vi "Unflatten Names.vi"   [LabVIEW 2020, in "SLSC.lvlib"]
doc: "Converts a comma-delimited list of names into an array of names. If the list contains colon-delimited ranges, they will be expanded."
uses:
  <vilib>/SLSC/SLSC.lvlib
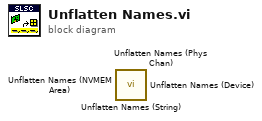
[diagram p0: block diagram]
diagram:
  n1 = call <vilib>:"Unflatten Names (String).vi"() -> ()  [unwired: 14 in, 2 out]
  n2 = call <vilib>:"Unflatten Names (Phys Chan).vi"() -> ()  [unwired: 14 in, 2 out]
  n3 = call <vilib>:"Unflatten Names (NVMEM Area).vi"() -> ()  [unwired: 14 in, 2 out]
  n4 = call <vilib>:"Unflatten Names (Device).vi"() -> ()  [unwired: 14 in, 2 out]
